vi "Initialize.vi"(4 "Ports":T1={"KA Port (9007)"=9007, "LtoP Port (9008)"=9008, "PtoL Port (9009)"=9009}, 5 "IP Address for LabVIEW Server":string, 7 "Server Alias":string, 8 "error in (no error)":errorcluster, 11 "VI Refnum":refnum<vi>) -> (0 "error out":errorcluster)   [LabVIEW 2013, in "TS.lvlib"]
doc: "This VI inits the main global variables, and dynamically runs the Server.vi."
uses:
  TS.lvlib
  LabVIEW Python Connector Message.ctl
  Private/Status Message.ctl
  Ports - Keep-Alive, LabVIEW-to-Python, Python-to-LabVIEW.ctl
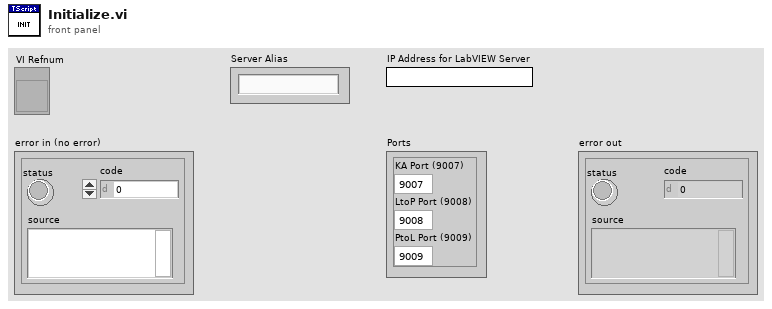
[diagram p1: front panel]
types:
  T1 = typedef "TS.lvlib/Ports - Keep-Alive, LabVIEW-to-Python, Python-to-LabVIEW.ctl" = cluster{"KA Port (9007)":u16, "LtoP Port (9008)":u16, "PtoL Port (9009)":u16}
  T2 = typedef "TS.lvlib/LabVIEW Python Connector Message.ctl" = cluster{"Command":string, "Data":string[], "Script ID":i64, "LabVIEW Server ID":string, "Python Message ID":i32}
  T3 = typedef "TS.lvlib/Status Message.ctl" = cluster{"Text":string, "Time":timestamp}
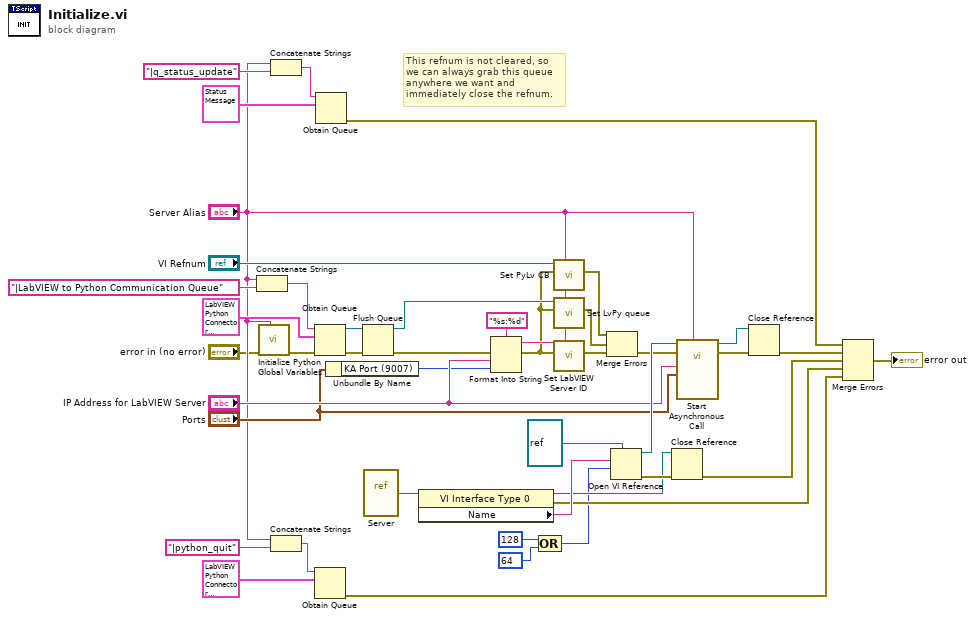
[diagram p0: block diagram]
diagram:
  # "This refnum is not cleared, so\nwe can always grab this queue\nanywhere we want and \nimmediately close the refnum."
  n1 = Concatenate Strings("Server Alias", "|LabVIEW to Python Communication Queue" ("name (unnamed)")) -> (w6:string)
  n2 = call "Initialize Python Global Variables.vi"("Server Alias"="Server Alias", "Error In"="error in (no error)") -> ("Error Out"=w1:errorcluster)  [unwired: 9 in]
  n3 = Concatenate Strings("Server Alias", "|q_status_update" ("name (unnamed)")) -> (w5:string)
  n4 = Concatenate Strings("Server Alias", "|python_quit" ("name (unnamed)")) -> (w7:string)
  n5 = Obtain Queue(name (unnamed)=w6, element data type=T2 {"Command"="zxcvbnm,", "Data"=["asdfghjk", "qwertyui"], "Script ID"=0, "LabVIEW Server ID"="zxcvbnm,", "Python Message ID"=0}, error in (no error)=w1) -> (queue out=w38:refnum<queue>, error out=w39:errorcluster)  [unwired: 2 in, 1 out]
  n6 = Obtain Queue(name (unnamed)=w7, element data type=T2 {"Command"="zxcvbnm,", "Data"=["asdfghjk", "qwertyui"], "Script ID"=0, "LabVIEW Server ID"="zxcvbnm,", "Python Message ID"=0}) -> (error out=w19:errorcluster)  [unwired: 3 in, 2 out]
  n7 = Obtain Queue(name (unnamed)=w5, element data type=T3 {"Text"="", "Time"=timestamp(0 s since 1904-01-01)} ("Status Update Message")) -> (error out=w31:errorcluster)  [unwired: 3 in, 2 out]
  n8 = Unbundle By Name("Ports") -> ("KA Port (9007)"=w16:u16)
  n9 = Flush Queue(queue=w38, error in (no error)=w39) -> (queue out=w36:refnum<queue>, error out=w35:errorcluster)  [unwired: 1 out]
  n10 = vi-ref "Server.vi"() -> (w30:refnum<vi>)
  n11 = property class="VI Interface Type 0"(reference=w30) -> (reference out=w29:refnum<vi>, error out=w27:errorcluster, "Name"=w41:string)  [unwired: 1 in]
  n12 = Format Into String(format string="%s:%d", error in=w35, "IP Address for LabVIEW Server", w16) -> (resulting string=w14:string, error out=w12:errorcluster)  [unwired: 1 in]
  n13 = Compound Arithmetic op=OR(128 ("options"), 64 ("options")) -> (w8:i32)
  n14 = call "Set PyLv CB.vi"("Server Alias"="Server Alias", "Error In"=w12, "VI Refnum"="VI Refnum") -> ("Error Out"=w10:errorcluster)  [unwired: 8 in]
  n15 = call "Set LvPy queue.vi"("Server Alias"="Server Alias", "Error In"=w12, "LvPy queue"=w36) -> ("Error Out"=w11:errorcluster)  [unwired: 8 in]
  n16 = call "Set LabVIEW Server ID.vi"("Server Alias"="Server Alias", "Error In"=w12, "LabVIEW Server ID"=w14) -> ("Error Out"=w13:errorcluster)  [unwired: 8 in]
  n17 = Merge Errors(w10, w11, w13) -> (w4:errorcluster)
  n18 = Open VI Reference(type specifier VI Refnum (for type only)=refnum<vi> refnum, vi path=w41, options=w8) -> (vi reference=w24:refnum<vi>, error out=w40:errorcluster)  [unwired: 3 in]
  n19 = Close Reference(reference=w29, error in (no error)=w40) -> (error out=w37:errorcluster)
  n20 = call-by-ref "Start Asynchronous Call"(reference=w24, error in=w4, "Server Alias"="Server Alias", "Ports"="Ports", "Local IP Address for LabVIEW Server"="IP Address for LabVIEW Server") -> (reference out=w22:refnum<vi>, error out=w23:errorcluster)  [unwired: 9 in]
  n21 = Close Reference(reference=w22, error in (no error)=w23) -> (error out=w28:errorcluster)
  n22 = Merge Errors(w31, w28, w37, w27, w19) -> (→"error out":errorcluster)
